vi "Offset_decompose.vi"(0 "DEC offset":dbl format="%.2f", 3 "RA offset":dbl format="%.2f", 4 "Micro Limit":dbl=2.0) -> (5 "Goffset":bool=TRUE, 6 "Moffset":bool, 7 "DEC Goffset":dbl format="%.2f", 8 "RA Goffset":dbl format="%.2f", 9 "DEC Moffset":dbl format="%.2f", 10 "RA Moffset":dbl format="%.2f")   [LabVIEW 2011]
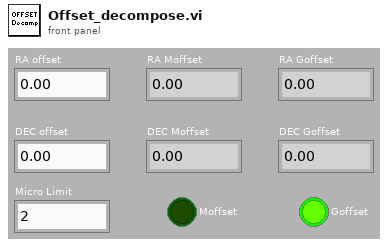
[diagram p1: front panel]
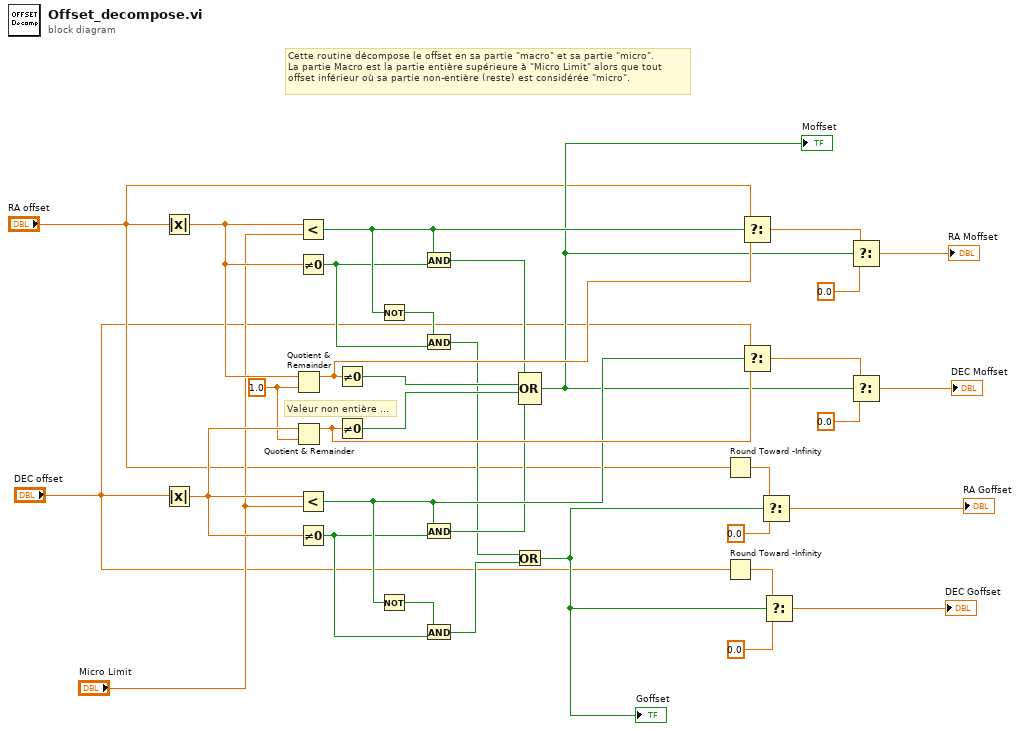
[diagram p0: block diagram]
diagram:
  w21 = 1.0 ("y")
  # "Cette routine décompose le offset en sa partie \"macro\" et sa partie \"micro\".\nLa partie Macro est la partie entière supérieure à \"Micro Limit\" alors que tout\noffset inférieur où sa partie non-entière (reste) est considérée \"micro\"."
  # "Valeur non entière ..."
  n1 = Absolute Value(x="RA offset") -> (abs(x)=w16:dbl)
  n2 = Absolute Value(x="DEC offset") -> (abs(x)=w22:dbl)
  n3 = Quotient & Remainder(x=w16, y=w21) -> (x-y*floor(x/y)=w28:dbl)  [unwired: 1 out]
  n4 = Quotient & Remainder(x=w22, y=w21) -> (x-y*floor(x/y)=w30:dbl)  [unwired: 1 out]
  n5 = Less?(x=w16, y="Micro Limit") -> (x < y?=w27:bool)
  n6 = Not Equal To 0?(x=w16) -> (x != 0?=w10:bool)
  n7 = Less?(x=w22, y="Micro Limit") -> (x < y?=w29:bool)
  n8 = Not Equal To 0?(x=w22) -> (x != 0?=w13:bool)
  n9 = Not Equal To 0?(x=w28) -> (x != 0?=w18:bool)
  n10 = Not Equal To 0?(x=w30) -> (x != 0?=w19:bool)
  n11 = Not(x=w27) -> (.not. x?=w11:bool)
  n12 = Not(x=w29) -> (.not. x?=w12:bool)
  n13 = And(x=w27, y=w10) -> (x .and. y?=w17:bool)
  n14 = And(x=w11, y=w10) -> (x .and. y?=w14:bool)
  n15 = And(x=w29, y=w13) -> (x .and. y?=w20:bool)
  n16 = And(x=w12, y=w13) -> (x .and. y?=w15:bool)
  n17 = Or(x=w14, y=w15) -> (x .or. y?=w8:bool)
  "Goffset" <- w8
  n18 = Compound Arithmetic op=OR(w17, w18, w19, w20) -> (w7:bool)
  "Moffset" <- w7
  n19 = Round Toward -Infinity(1:"RA offset") -> (0:w24:dbl)
  n20 = Round Toward -Infinity(1:"DEC offset") -> (0:w23:dbl)
  n21 = Select(t="RA offset", s=w27, f=w28) -> (s? t:f=w32:dbl)
  n22 = Select(t="DEC offset", s=w29, f=w30) -> (s? t:f=w31:dbl)
  n23 = Select(t=w24, s=w8, f=0.0) -> (s? t:f=→"RA Goffset":dbl)
  n24 = Select(t=w23, s=w8, f=0.0) -> (s? t:f=→"DEC Goffset":dbl)
  n25 = Select(t=w32, s=w7, f=0.0) -> (s? t:f=→"RA Moffset":dbl)
  n26 = Select(t=w31, s=w7, f=0.0) -> (s? t:f=→"DEC Moffset":dbl)
